vi "VESASignal_ScanNextHPixel.vi"() -> (15 "h_Pixel":i16, 17 "Enable":bool)   [LabVIEW 2018]
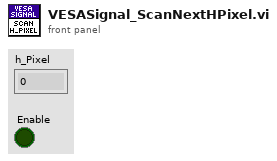
[diagram p1: front panel]
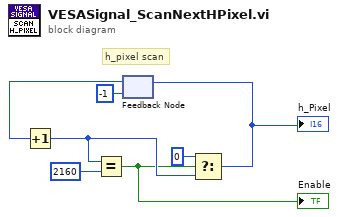
[diagram p0: block diagram]
diagram:
  # "h_pixel scan"
  n1 = feedback #1(i16 -1 ("f")) -> (w7:i16)
  n2 = Increment(x=w7) -> (x+1=w5:i16)
  n3 = Equal?(x=w5, y=i16 2160) -> (x = y?=w2:bool)
  "Enable" <- w2
  n4 = Select(t=i16 0 ("f"), s=w2, f=w5) -> (s? t:f=w3:i16)
  "h_Pixel" <- w3
  n5 = feedback-in #1(w3) -> ()
